vi "GV RS edge.vi"() -> ()   [LabVIEW 2017]
panel:
  out "RS edge":bool
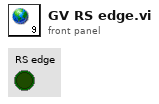
[diagram p1: front panel]
diagram:
